vi "FTW-Endpoint-Bind.vi"(0 "FTW ØMQ Endpoint":refnum<class "FTW-Endpoint-ZMQ.lvclass">, 5 "Endpoint Address":T1, 7 "Requested Identity":string, 11 "error in":errorcluster) -> (4 "FTW ØMQ Endpoint out":refnum<class "FTW-Endpoint-ZMQ.lvclass">, 6 "Actual Endpoint Address":T1, 8 "Actual Identity":string, 15 "error out":errorcluster)   [LabVIEW 2012, in "FTW-Actor.lvlib" / "FTW-Endpoint-ZMQ.lvclass"]
uses:
  FTW-Endpoint-ZMQ.lvclass
  Utility/FTW-Actor-Address.ctl
  FTW-Endpoint-ZMQ.lvclass/FTW-Endpoint-ZMQ.ctl
  FTW-Actor.lvlib
panel:
  # "Inputs"
  # "Outputs"
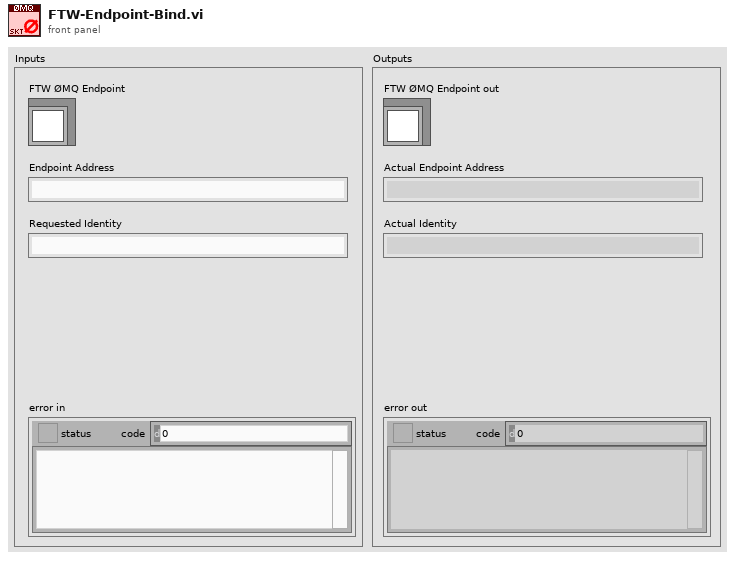
[diagram p1: front panel]
types:
  T1 = typedef "FTW-Actor.lvlib/FTW-Actor-Address.ctl" = string
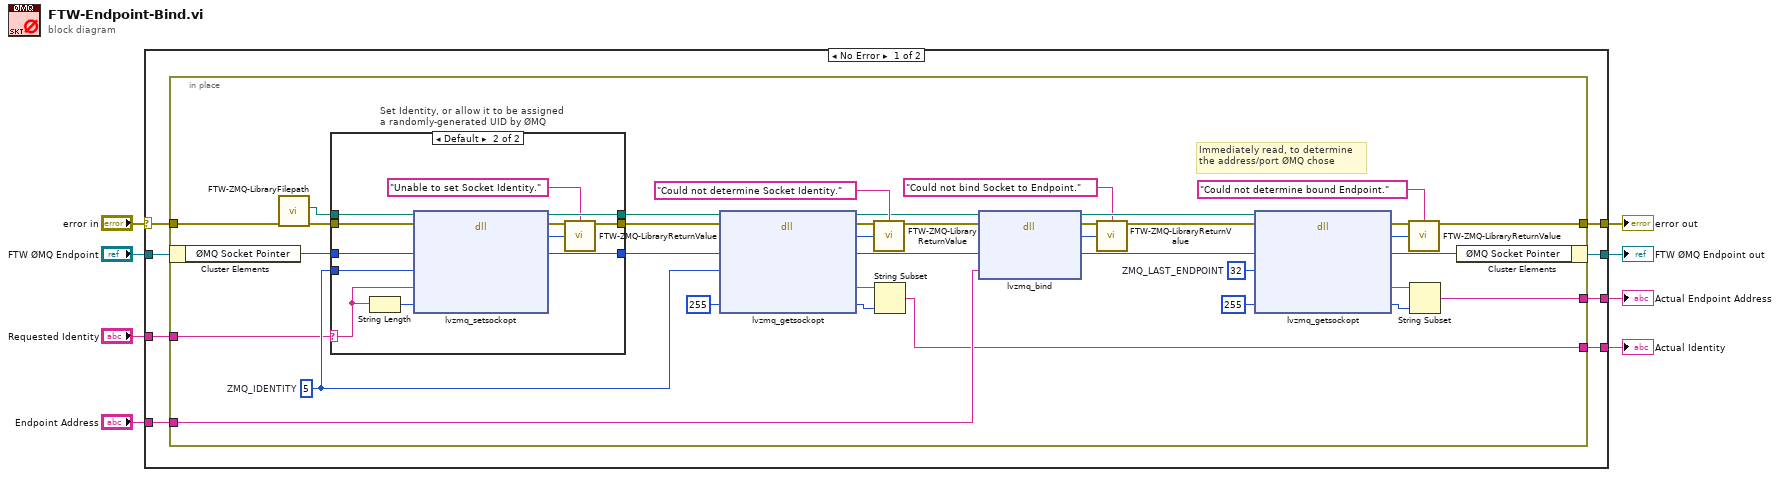
[diagram p0: block diagram]
diagram:
  n1 = case shown="No Error" "error in" {
    selector: "error in" -> [w9 w68]
    tunnel: "FTW ØMQ Endpoint" -> [w11 w69]
    tunnel: [w13 w68] -> w7
    tunnel: [w16 w69] -> w6
    tunnel: "Endpoint Address" -> [w15 _]
    tunnel: [w14 _] -> w3
    tunnel: "Requested Identity" -> [w10 _]
    tunnel: [w12 _] -> w1
    frame No Error {
      n2 = in-place {
        in-place-border: w9 -> [w24]
        in-place-border: w15 -> [w52]
        in-place-border: [w51] -> w14
        in-place-border: [w37] -> w13
        in-place-border: [w23] -> w12
        in-place-border: w10 -> [w22]
        w35 = 5  # ZMQ_IDENTITY
        w47 = 32  # ZMQ_LAST_ENDPOINT
        # "Immediately read, to determine\nthe address/port ØMQ chose"
        n3 = in-place-cluster #1(w11) -> ("ØMQ Socket Pointer"=w20:u64)
        n4 = call "FTW-ZMQ-LibraryFilepath.vi"("error in"=w24) -> ("error out"=w21:errorcluster, "FTW-ZMQ Library Filepath"=w25:path)  [unwired: 8 in, 1 out]
        n5 = case "Set Identity, or allow it to be assigned\na randomly-generated UID by ØMQ" shown="Default" w22 {
          selector: w22 -> [_ w61]
          tunnel: w21 -> [w54 w67]
          tunnel: w25 -> [w55 w65]
          tunnel: [w55 w64] -> w31
          tunnel: [w53 w63] -> w29
          tunnel: w20 -> [w53 w62]
          tunnel: [w54 w58] -> w30
          tunnel: w35 -> [_ w60]
          frame "" {
          }
          frame Default {
            n6 = String Length(string=w61) -> (length=w66:i32)
            n7 = dll-call lib="?" fn="lvzmq_setsockopt"(path in=w65, error in=w67, "Socket Pointer"=w62, "Socket Option"=w60, "Option Value"=w61, "Option Value Length"=w66) -> (path out=w64:path, error out=w59:errorcluster, "Return Value"=w57:i32, "Socket Pointer"=w63:u64)  [unwired: 4 in]
            n8 = call "FTW-ZMQ-LibraryReturnValue.vi"("error in"=w59, "Error Message"="Unable to set Socket Identity.", "Return Value"=w57) -> ("error out"=w58:errorcluster)  [unwired: 12 in]
          }
        }
        n9 = dll-call lib="?" fn="lvzmq_getsockopt"(path in=w31, error in=w30, "Socket Pointer"=w29, "Socket Option"=w35, "Option Value Length"=u32 255) -> (path out=w18:path, error out=w27:errorcluster, "Return Value"=w26:i32, "Socket Pointer"=w19:u64, "Option Value"=w33:string, "Option Value Length"=w32:u32)  [unwired: 3 in]
        n10 = call "FTW-ZMQ-LibraryReturnValue.vi"("error in"=w27, "Error Message"="Could not determine Socket Identity.", "Return Value"=w26) -> ("error out"=w17:errorcluster)  [unwired: 12 in]
        n11 = String Subset(string=w33, length (rest)=w32) -> (substring=w23:string)  [unwired: 1 in]
        n12 = dll-call lib="?" fn="lvzmq_bind"(path in=w18, error in=w17, "Socket Pointer"=w19, "Endpoint"=w52) -> (path out=w46:path, error out=w44:errorcluster, "Return Value"=w43:i32, "Socket Pointer"=w45:u64)  [unwired: 2 in]
        n13 = call "FTW-ZMQ-LibraryReturnValue.vi"("error in"=w44, "Error Message"="Could not bind Socket to Endpoint.", "Return Value"=w43) -> ("error out"=w42:errorcluster)  [unwired: 12 in]
        n14 = dll-call lib="?" fn="lvzmq_getsockopt"(path in=w46, error in=w42, "Socket Pointer"=w45, "Socket Option"=w47, "Option Value Length"=u32 255) -> (error out=w40:errorcluster, "Return Value"=w39:i32, "Socket Pointer"=w36:u64, "Option Value"=w49:string, "Option Value Length"=w50:u32)  [unwired: 3 in, 1 out]
        n15 = call "FTW-ZMQ-LibraryReturnValue.vi"("error in"=w40, "Error Message"="Could not determine bound Endpoint.", "Return Value"=w39) -> ("error out"=w37:errorcluster)  [unwired: 12 in]
        n16 = String Subset(string=w49, length (rest)=w50) -> (substring=w51:string)  [unwired: 1 in]
        n17 = in-place-cluster #1("ØMQ Socket Pointer"=w36) -> (w16:refnum<class "FTW-Endpoint-ZMQ.lvclass">)
      }
    }
    frame Error {
    }
  }
  "error out" <- w7
  "FTW ØMQ Endpoint out" <- w6
  "Actual Endpoint Address" <- w3
  "Actual Identity" <- w1
